vi "check power fifo load.vi"(11 "Refnum in":T1) -> (1 "ready":bool, 3 "Power measurements Remaining":u32)   [LabVIEW 2020]
uses:
  Host/SubVIs/Streaming Xvcr FPGA Ref.ctl
  <vilib>/Utility/error.llb/Error Cluster From Error Code.vi
  <vilib>/rvi/errors/niLvFpgaAdjustHostInterfaceError.vi
  <vilib>/rvi/interface/nirviMethod/nirviMethod.xnode
  <vilib>/FPGAPlugInAG/Dynamic/niLvFpga_ReadFifo_Dynamic.vi
  <vilib>/rvi/errors/niLvFpgaMergeErrorWithErrorCode.vi
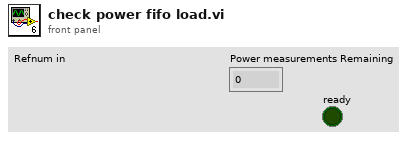
[diagram p1: front panel]
types:
  T1 = typedef "Streaming Xvcr FPGA Ref.ctl" = refnum<k20>
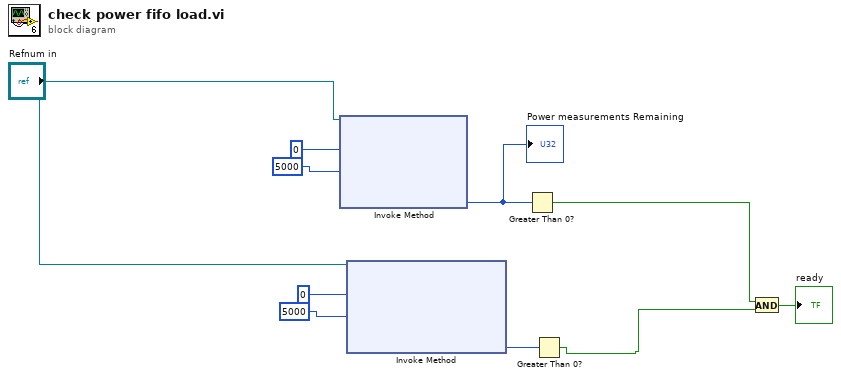
[diagram p0: block diagram]
diagram:
  n1 = xnode "Invoke Method"("FPGA VI Reference In"="Refnum in", "Number of Elements"=u32 0, "Timeout (ms)"=5000) -> ("Elements Remaining"=w6:u32)  [unwired: 1 in, 3 out]
  "Power measurements Remaining" <- w6
  n2 = xnode "Invoke Method"("FPGA VI Reference In"="Refnum in", "Number of Elements"=u32 0, "Timeout (ms)"=5000) -> ("Elements Remaining"=w9:u32)  [unwired: 1 in, 3 out]
  n3 = Greater Than 0?(x=w6) -> (x > 0?=w2:bool)
  n4 = Greater Than 0?(x=w9) -> (x > 0?=w3:bool)
  n5 = And(x=w2, y=w3) -> (x .and. y?=→"ready":bool)
